vi "Drive Tank.vi"(8 "error in":errorcluster, 9 "Force? (F)":bool, 10 "Right":dbl, 11 "Left":dbl) -> (0 "error out":errorcluster)   [LabVIEW 2016, in "Drive System.lvlib"]
uses:
  Drive System.lvlib
  Private/DriveCmd.ctl
  Private/DriveCmdList.ctl
  Private/Varient Cmd Types/Drive Tank.ctl
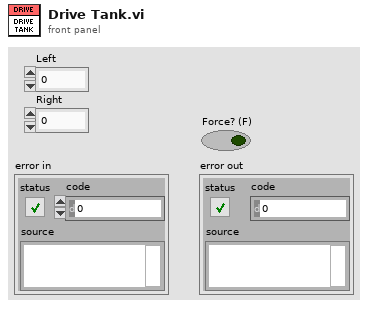
[diagram p1: front panel]
types:
  T1 = typedef "Drive System.lvlib/Drive Tank.ctl" = cluster{"Left":dbl, "Right":dbl}
  T2 = typedef "Drive System.lvlib/DriveCmd.ctl" = cluster{"cmd":T3, "data":variant, "Force? (F)":bool}
  T3 = typedef "Drive System.lvlib/DriveCmdList.ctl" = enum16{"Cleanup", "Drive For Time", "Drive Tank", "Drive Arcade", "Unlock", "Lock"}
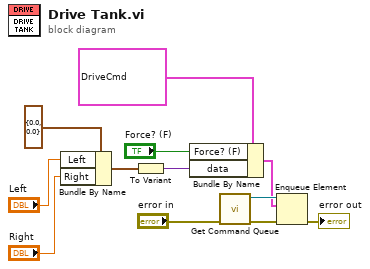
[diagram p0: block diagram]
diagram:
  n1 = Bundle By Name(cluster=T1 {"Left"=0.0, "Right"=0.0} ("Cluster"), "Left"="Left", "Right"="Right") -> (w6:T1)
  n2 = To Variant(anything=w6) -> (Variant=w5:variant)
  n3 = Bundle By Name(cluster=T2 {"cmd"=enum."Drive Tank", "data"=variant, "Force? (F)"=FALSE} ("element"), "Force? (F)"="Force? (F)", "data"=w5) -> (w2:T2)
  n4 = call "Get Command Queue.vi"("error in (no error)"="error in") -> ("error out"=w10:errorcluster, "Queue out"=w9:refnum<queue>)  [unwired: 9 in]
  n5 = Enqueue Element(queue=w9, element=w2, error in (no error)=w10) -> (error out=→"error out":errorcluster)  [unwired: 1 in, 2 out]
